vi "close.vi"(8 "error in (no error)":errorcluster caption="错误输入（无错误）", 11 "LXMCU_40G_HUAWEI 输入":refnum<class "LXMCU_40G_HUAWEI.lvclass"> caption="DNL_LabVIEW Object in") -> (0 "error out":errorcluster caption="错误输出", 3 "LXMCU_40G_HUAWEI 输出":refnum<class "LXMCU_40G_HUAWEI.lvclass"> caption="DNL_LabVIEW Object out")   [LabVIEW 2011, in "LXMCU_40G_HUAWEI.lvclass"]
uses:
  LXMCU_40G_HUAWEI.lvclass
  LXMCU_40G_HUAWEI.lvclass/LXMCU_40G_HUAWEI.ctl
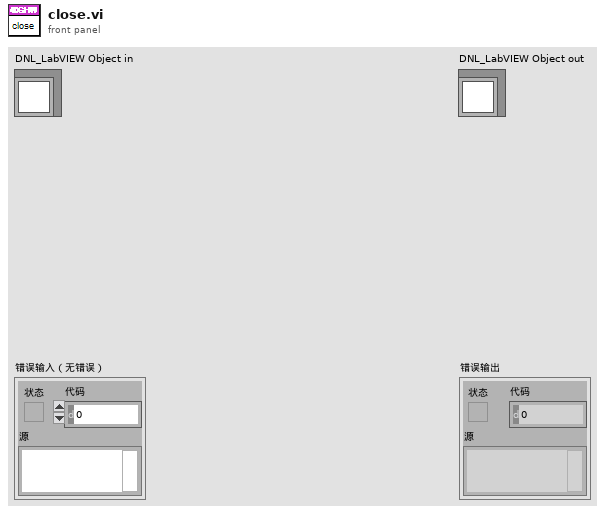
[diagram p1: front panel]
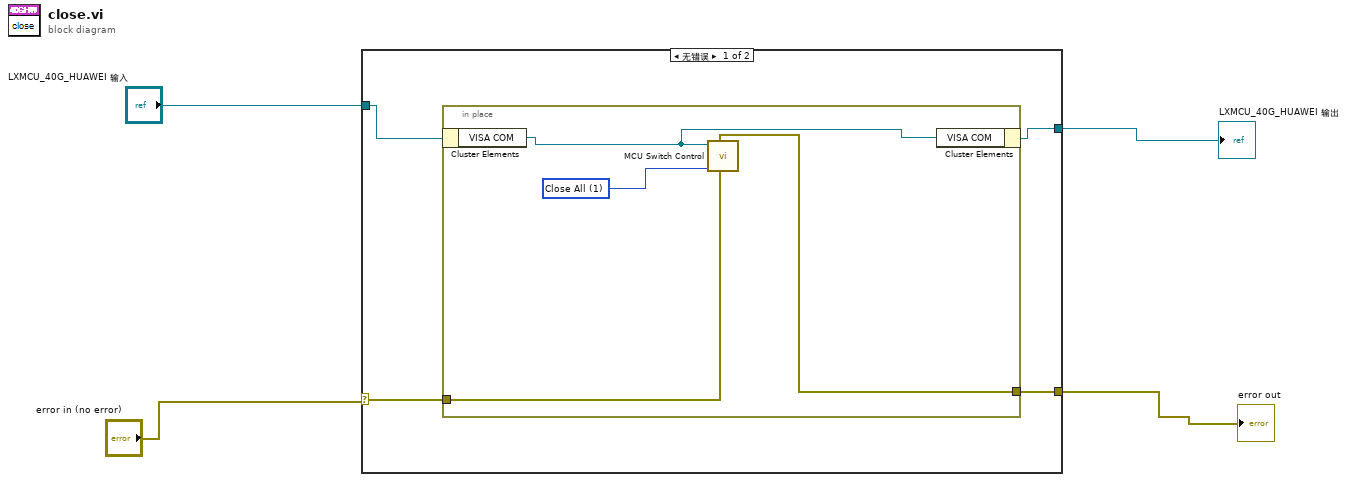
[diagram p0: block diagram]
diagram:
  n1 = case shown="无错误" "error in (no error)" {
    selector: "error in (no error)" -> [w7 w13]
    tunnel: "LXMCU_40G_HUAWEI 输入" -> [w8 w14]
    tunnel: [w6 w14] -> w3
    tunnel: [w5 w13] -> w2
    frame No Error {
      n2 = in-place {
        in-place-border: w7 -> [w11]
        in-place-border: [w10] -> w5
        w12 = u16 1 items=["Testing", "Close All"] ("Function")
        n3 = in-place-cluster #1(w8) -> ("VISA COM"=w9:refnum<visa-resource-name>)
        n4 = call "MCU Switch Control.vi"("Error in"=w11, "Function"=w12, "VISA"=w9) -> ("error out"=w10:errorcluster)  [unwired: 8 in]
        n5 = in-place-cluster #1("VISA COM"=w9) -> (w6:refnum<class "LXMCU_40G_HUAWEI.lvclass">)
      }
    }
    frame Error {
    }
  }
  "error out" <- w2
  "LXMCU_40G_HUAWEI 输出" <- w3
